vi "Build Axis Indicators.vi"(8 "Error In":errorcluster, 9 "Sample Period":dbl, 10 "Sample Freq.":dbl, 11 "Axis Pos.":dbl[](array[numeric])) -> (0 "Error Out":errorcluster, 3 "Axis Inds. out":T1)   [LabVIEW 2013]
doc: "This sub-VI takes an array of axis positions and bundles them into the axis indicators cluster. It also filters\nthe axis positions to avoid excessively large fluctuations due to bad position reads, and determines whether\nan axis is moving."
uses:
  Controls/axis_indicator_cluster.ctl
  <vilib>/Analysis/_algsub.llb/Vector Norm Type.ctl
  <vilib>/Analysis/_algsub.llb/Real Vector Norm.vi
  <vilib>/ptbypt/NI_PtbyPt.lvlib
  <vilib>/Analysis/NI_AALPro.lvlib
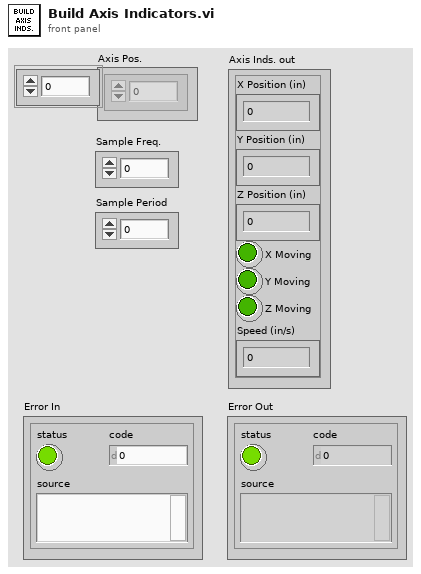
[diagram p1: front panel]
types:
  T1 = typedef "axis_indicator_cluster.ctl" = cluster{"X Position (in)":dbl, "Y Position (in)":dbl, "Z Position (in)":dbl, "X Moving":bool, "Y Moving":bool, "Z Moving":bool, "Speed (in/s)":dbl}
  T2 = typedef "NI_AALPro.lvlib/Vector Norm Type.ctl" = u16
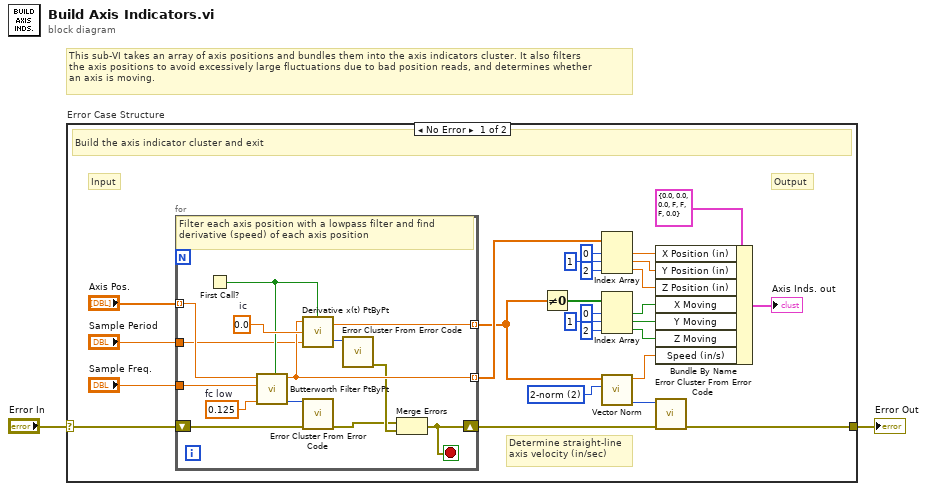
[diagram p0: block diagram]
diagram:
  # "This sub-VI takes an array of axis positions and bundles them into the axis indicators cluster. It also filters\nthe axis positions to avoid excessively large fluctuations due to bad position reads, and determines whether\nan axis is moving."
  n1 = case "Error Case Structure" shown="No Error" "Error In" {
    selector: "Error In" -> [w20 w43]
    tunnel: [w8 w43] -> w1
    frame No Error {
      w3 = T2 2 items=["1-norm"=1, "2-norm"=2, "Inf-norm"=3, "-Inf-norm"=4, "User Defined"=5] ("norm type")
      # "Determine straight-line\naxis velocity (in/sec)"
      # "Output"
      # "Input"
      # "Build the axis indicator cluster and exit"
      n2 = for {
        tunnel: "Axis Pos." -> [w38] mode=indexing
        tunnel: [w32] -> w17 mode=indexing
        shift-right: [w33] -> w9
        shift-left: w20 -> [w42]
        tunnel: "Sample Freq." -> [w40]
        tunnel: "Sample Period" -> [w29]
        tunnel: [w35] -> w5 mode=indexing
        stop <- w33 stop-if-true
        w37 = 0.0  # ic
        w39 = 0.125  # fc low
        # "Filter each axis position with a lowpass filter and find derivative (speed) of each axis position"
        n3 = First Call?() -> (First Call?: T/F=w34:bool)
        n4 = call <vilib>:"Butterworth Filter PtByPt.vi"("initialize"=w34, "low cutoff freq: fl"=w39, "sampling freq: fs"=w40, "x"=w38) -> ("error"=w41:i32, "Filtered x"=w32:dbl)  [unwired: 5 in]
        n5 = call <vilib>:"Derivative x(t) PtByPt.vi"("initialize"=w34, "dt"=w29, "initial condition"=w37, "x"=w32) -> ("error"=w36:i32, "dx/dt"=w35:dbl)
        n6 = call <vilib>:"Error Cluster From Error Code.vi"("error in (no error)"=w42, "error code (0)"=w41) -> ("error out"=w30:errorcluster)  [unwired: 7 in]
        n7 = call <vilib>:"Error Cluster From Error Code.vi"("error code (0)"=w36) -> ("error out"=w31:errorcluster)  [unwired: 8 in]
        n8 = Merge Errors(w30, w31) -> (w33:errorcluster)
      }
      n9 = Not Equal To 0?(x=w5) -> (x != 0?=w4:bool[])
      n10 = Index Array(array=w17, index #1=0 ("index"), index #2=1 ("index"), index #3=2 ("index")) -> (element #1=w26:dbl, element #2=w27:dbl, element #3=w28:dbl)
      n11 = Index Array(array=w4, index #1=0 ("index"), index #2=1 ("index"), index #3=2 ("index")) -> (element #1=w13:bool, element #2=w12:bool, element #3=w6:bool)
      n12 = call-poly <vilib>:"Vector Norm.vi"("norm type"=w3, "Input Vector"=w5) -> ("error"=w7:i32, "norm"=w10:dbl)  [unwired: 8 in]
      n13 = Bundle By Name(cluster=T1 {"X Position (in)"=0.0, "Y Position (in)"=0.0, "Z Position (in)"=0.0, "X Moving"=FALSE, "Y Moving"=FALSE, "Z Moving"=FALSE, "Speed (in/s)"=0.0} ("Axis Inds. 2"), "X Position (in)"=w26, "Y Position (in)"=w27, "Z Position (in)"=w28, "X Moving"=w13, "Y Moving"=w12, "Z Moving"=w6, "Speed (in/s)"=w10) -> (→"Axis Inds. out":T1)
      n14 = call <vilib>:"Error Cluster From Error Code.vi"("error in (no error)"=w9, "error code (0)"=w7) -> ("error out"=w8:errorcluster)  [unwired: 7 in]
    }
    frame Error {
      # "Pass through and exit"
    }
  }
  "Error Out" <- w1
